vi "7. CoffeeMaker User Selection.vi"() -> ()   [LabVIEW 2018]
doc: "Coffee Machine Version 1.0: reacting correctly on user selections"
uses:
  Controls/States.ctl
  <vilib>/Utility/miscctls.llb/LVMinMaxIncTypeDef.ctl
  <vilib>/Utility/file.llb/Read Delimited Spreadsheet (string).vi
panel:
  out "s? t:f":enum16{"next state", "current state"}(ring)
  out "error out":errorcluster
  in  "error in (no error)":errorcluster
  in  "Power Switch":bool
  in  "Simulation":cluster{"Water":dbl, "Coffee":dbl, "Milk":dbl} caption="Wasser" {"Milk" scale=0.0..100.0; "Water" scale=0.0..100.0; "Coffee" scale=0.0..100.0}
  out "Display":T1 {"Coffee" scale=0.0..80.0; "Brewing Chamber" scale=0.0..80.0}
  in  "Coffee Selection":T2 {"Type" min=0 max=0 step=1 scale=0.0..2.0}
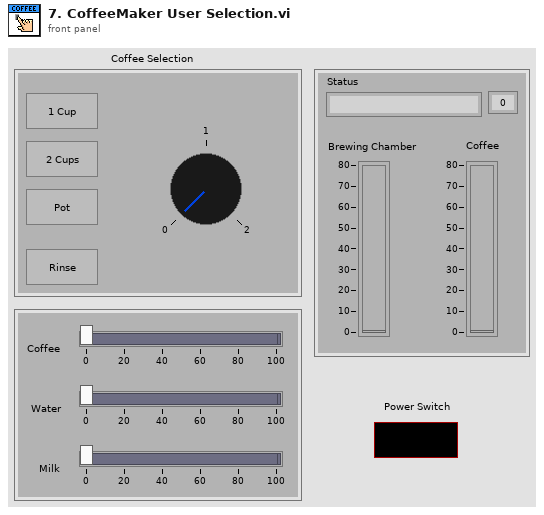
[diagram p1: front panel]
types:
  T1 = cluster{"Brewing Chamber":dbl, "Coffee":dbl, "Status":string, "Remaining Time:":i32}
  T2 = cluster{"1 Cup":bool, "2 Cups":bool, "Pot":bool, "Rinse":bool, "Type":i8}
  T3 = cluster{"Status":refnum<vi>, "Brewing Chamber":refnum<vi>, "Coffee":refnum<vi>, "Power Switch":refnum<vi>}
  T4 = enum8{"Enabled", "Disabled", "Disabled and Grayed Out"}
  T5 = typedef "LVMinMaxIncTypeDef.ctl" = cluster{"Minimum":dbl, "Maximum":dbl, "Increment":dbl}
  T6 = typedef "States.ctl" = enum16{"Initialize", "Set Language", "Wait for Power On", "Heat up", "Check and Wait for Water", "Rinsing", "Check Resources", "User Input", "Grinding", "Boiling", "Pouring", "Rinse before Stop", "Write Data", "Stop"}
  T7 = cluster{"Coffee":refnum<vi>, "Water":refnum<vi>, "Milk":refnum<vi>}
  T8 = cluster{"Coffee Selection":refnum<vi>, "1 Cup":refnum<vi>, "2 Cups":refnum<vi>, "Pot":refnum<vi>, "Rinse":refnum<vi>, "Type":refnum<vi>}
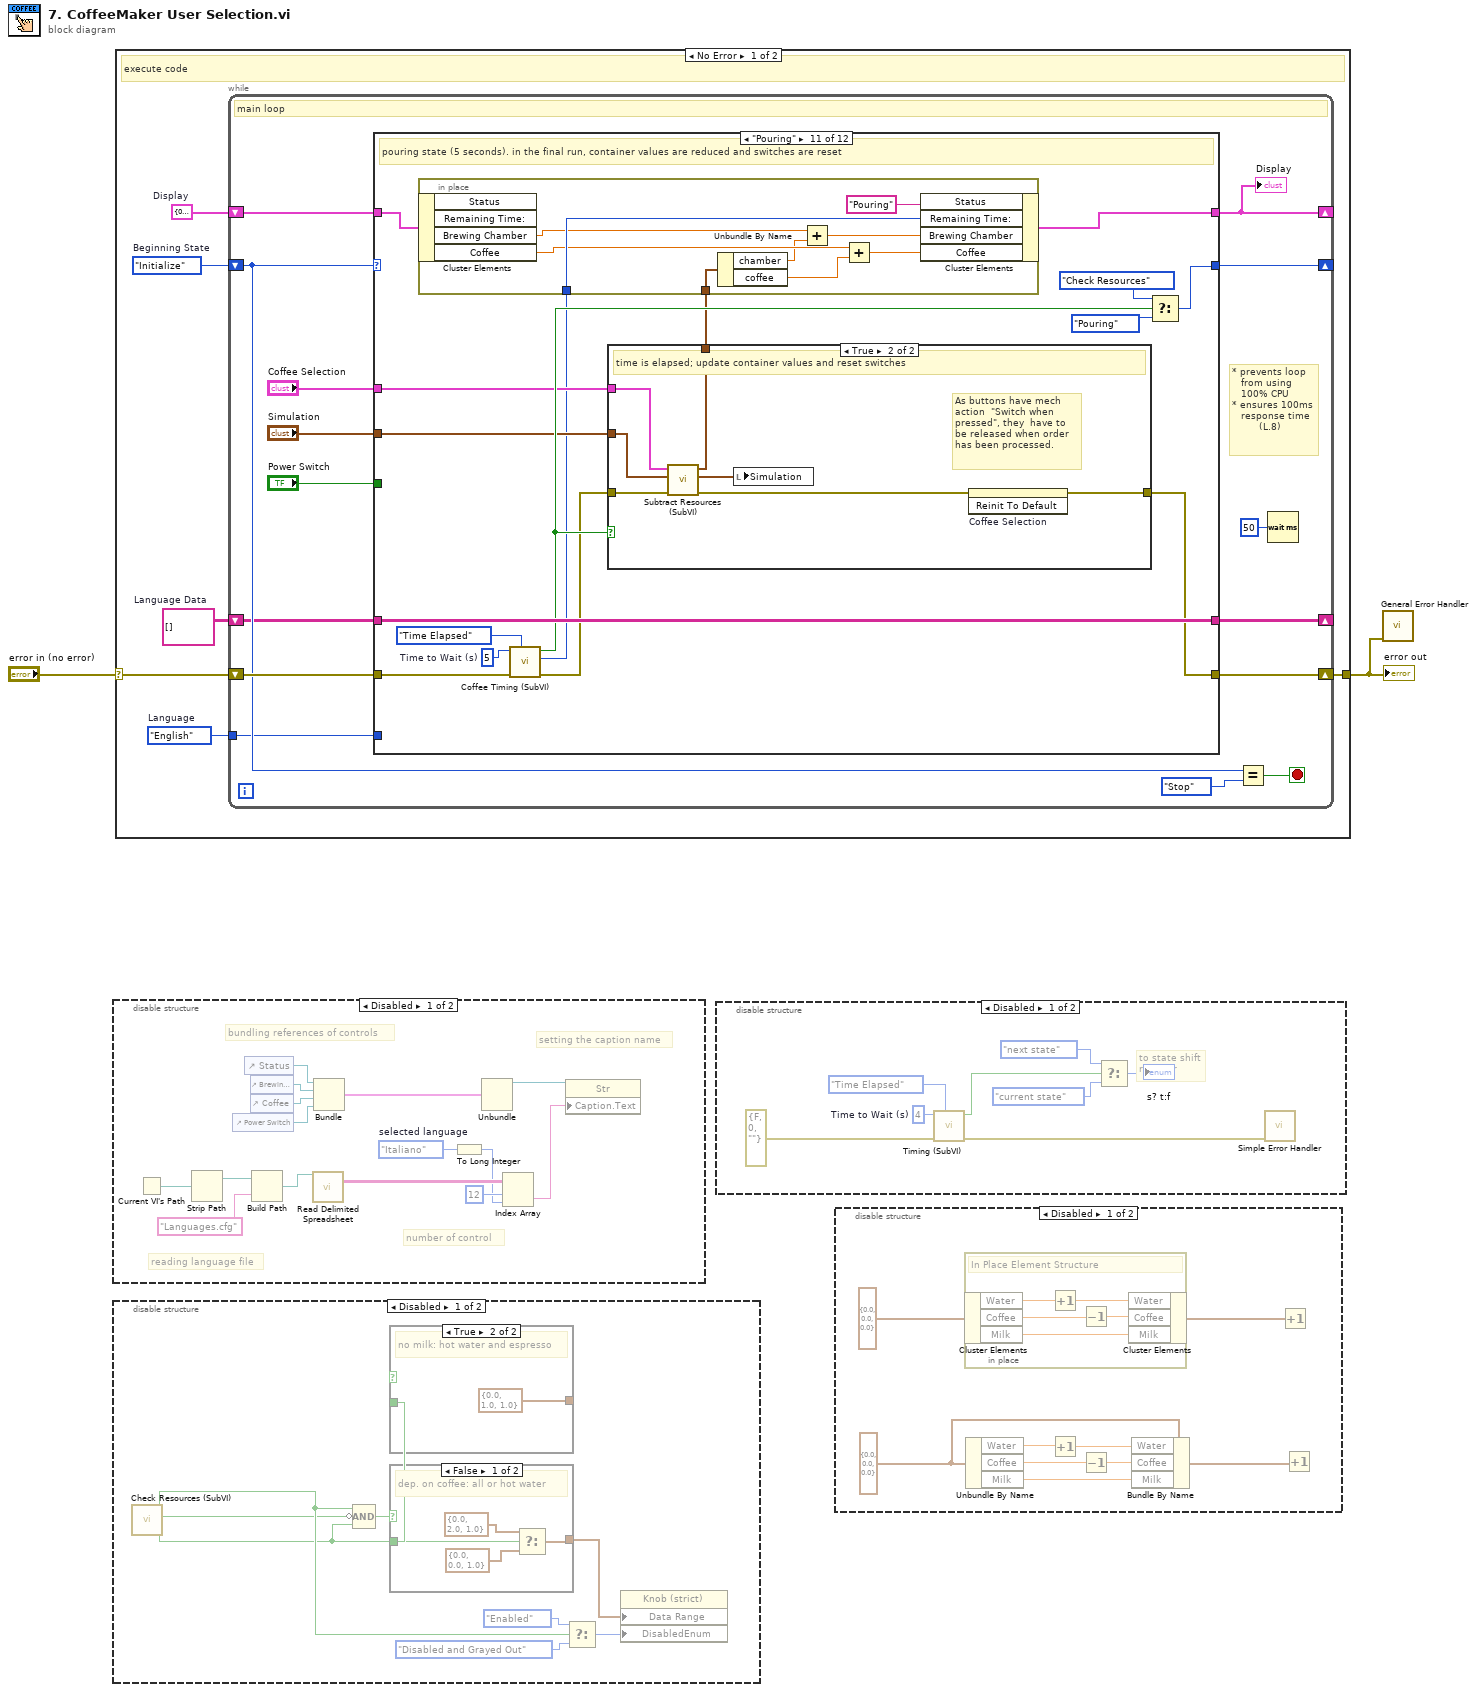
[diagram p0: block diagram]
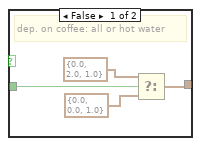
[diagram p3: hidden frame]
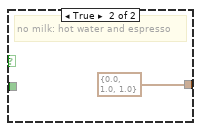
[diagram p4: hidden frame]
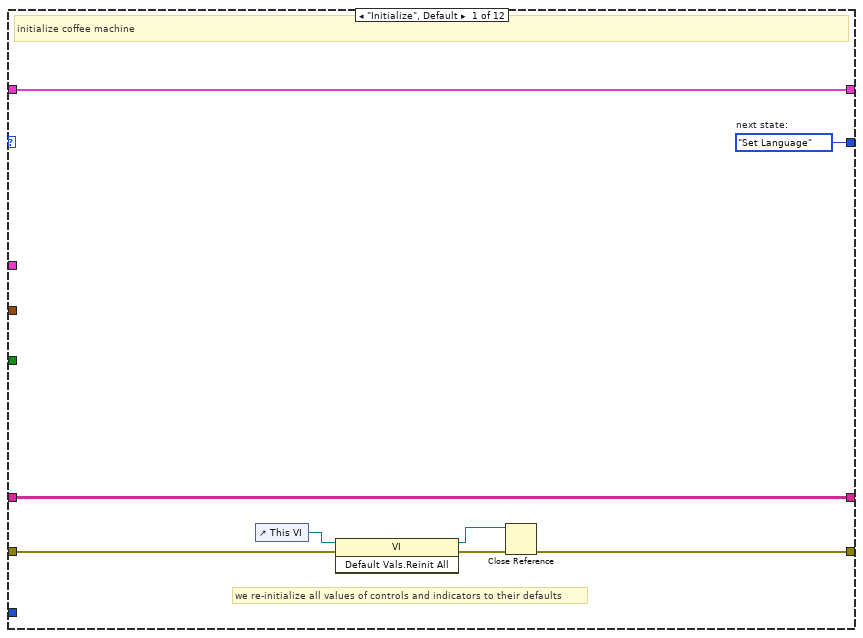
[diagram p8: hidden frame]
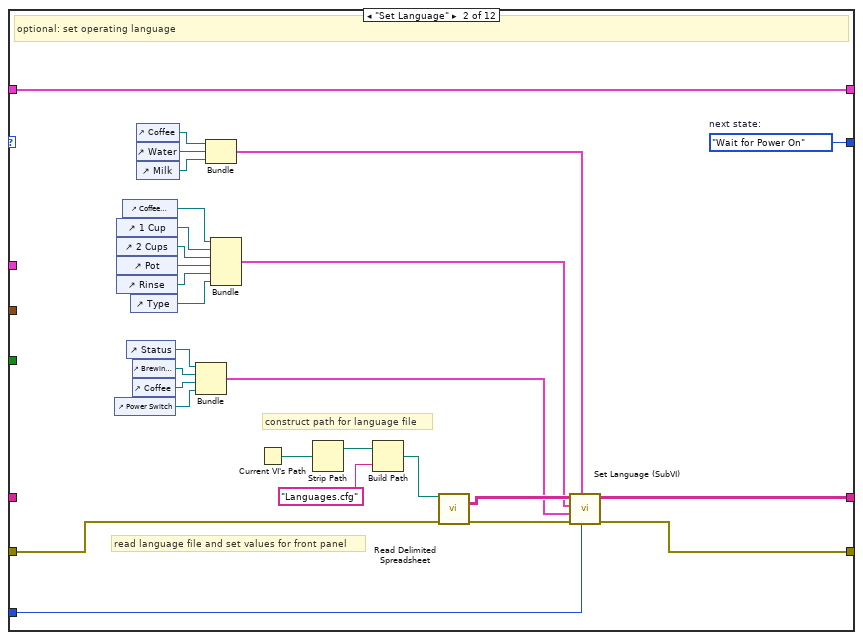
[diagram p9: hidden frame]
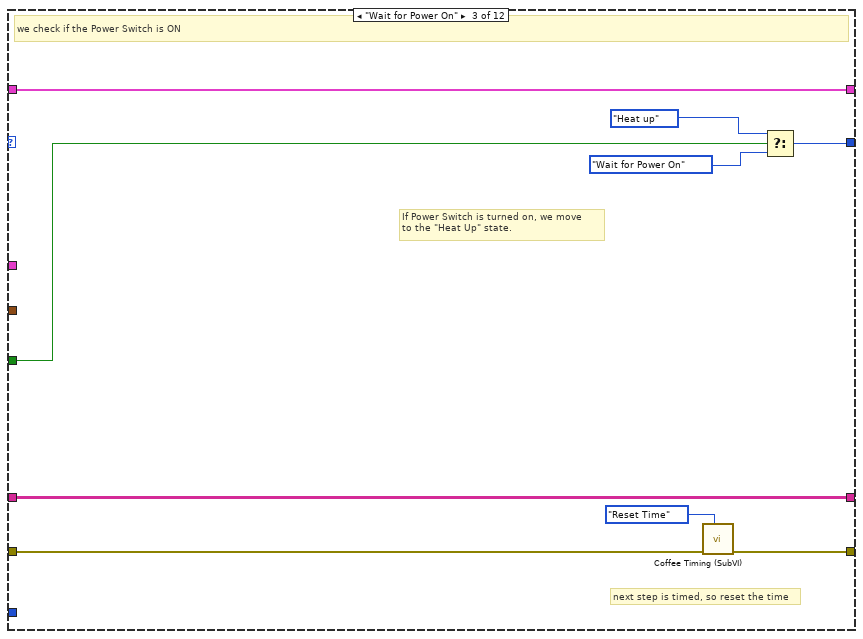
[diagram p10: hidden frame]
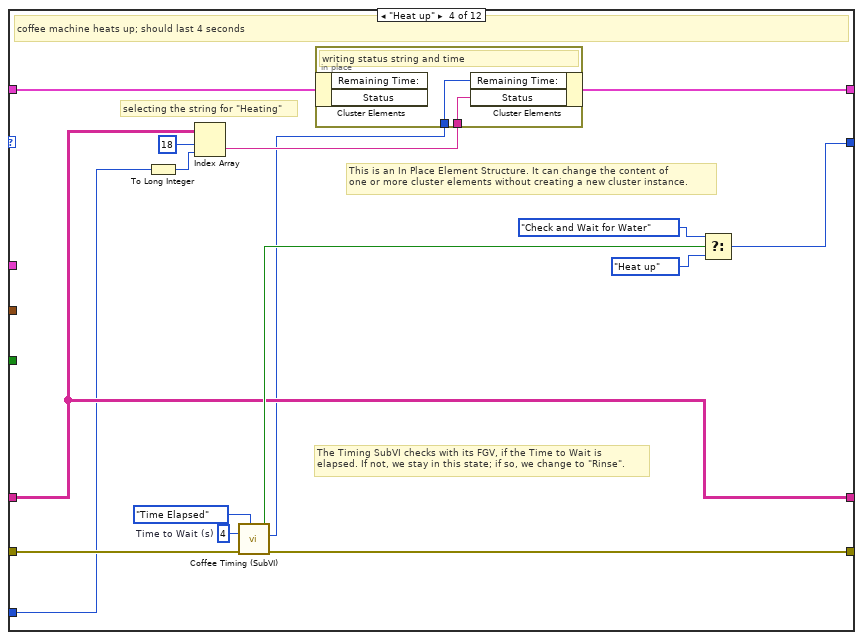
[diagram p11: hidden frame]
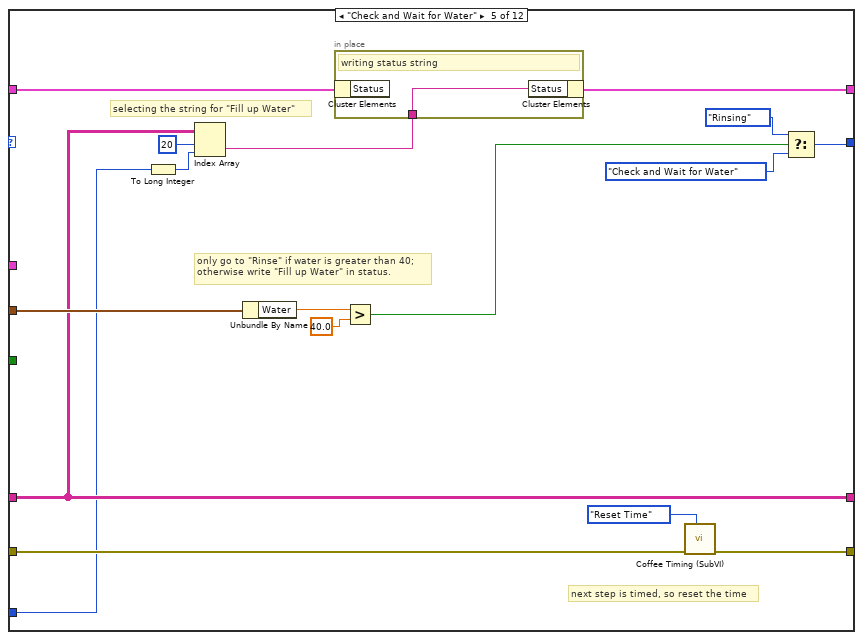
[diagram p12: hidden frame]
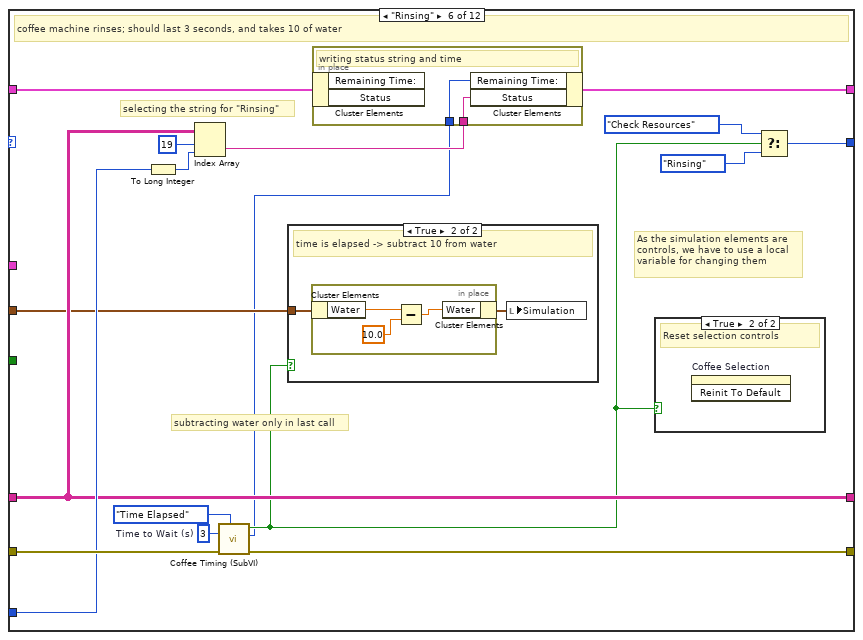
[diagram p13: hidden frame]
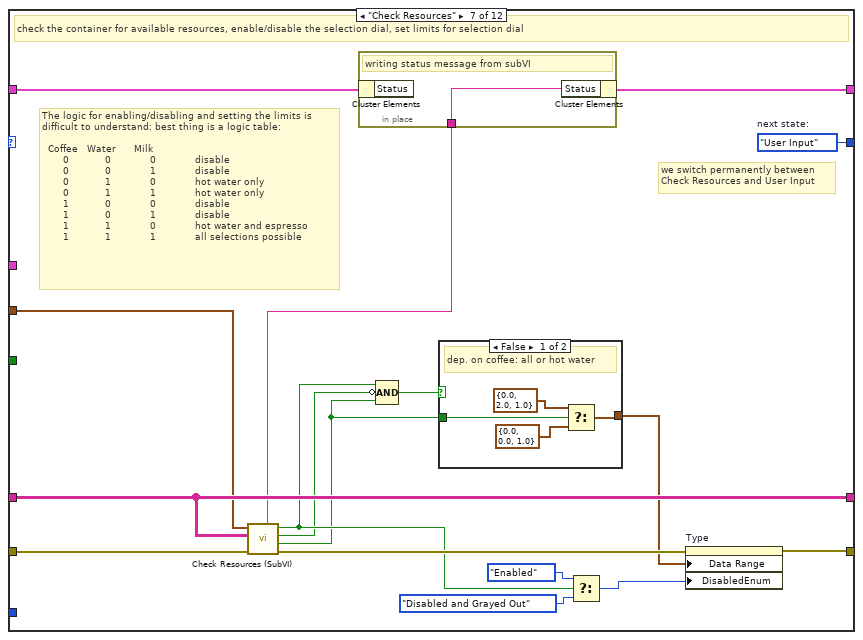
[diagram p16: hidden frame]
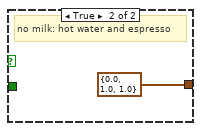
[diagram p17: hidden frame]
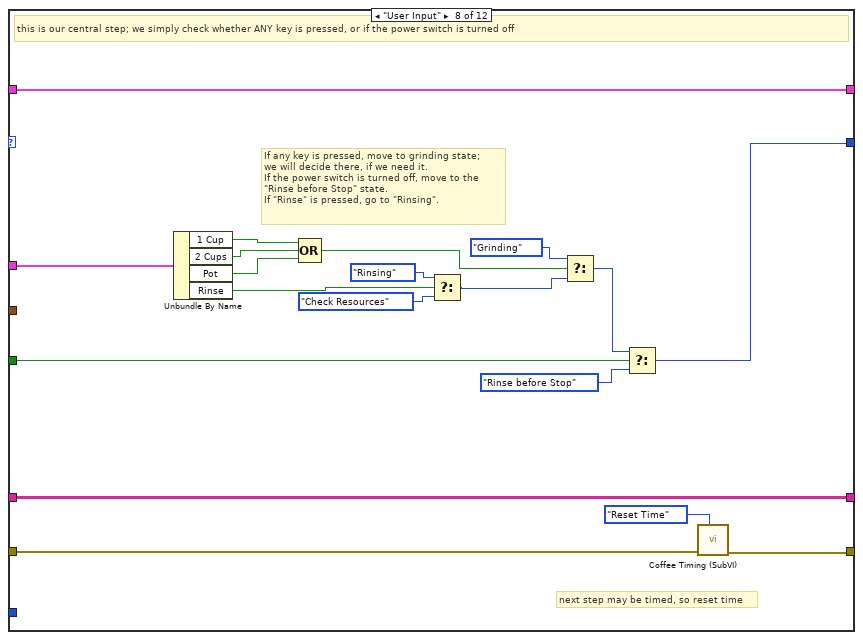
[diagram p18: hidden frame]
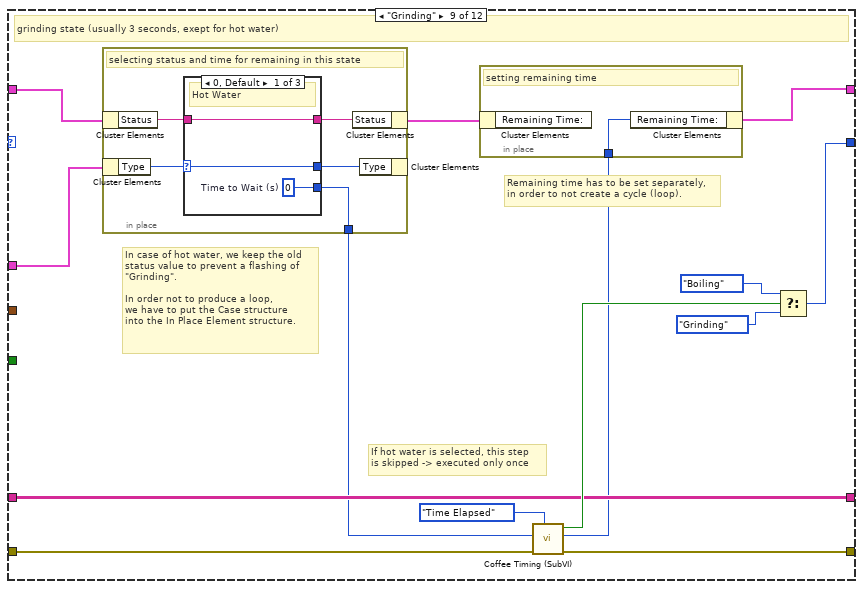
[diagram p19: hidden frame]
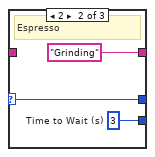
[diagram p20: hidden frame]
diagram:
  n1 = disable-structure shown="Disabled" {
    frame Disabled {
      w5 = enum16{"English", "Deutsch", "Italiano"}."Italiano"  # selected language
      # "setting the caption name"
      # "number of control"
      # "reading language file"
      # "bundling references of controls"
      n2 = Current VI's Path() -> (path=w11:path)
      n3 = Strip Path(path=w11) -> (stripped path=w10:path)  [unwired: 1 out]
      n4 = control-ref of="Power Switch"() -> (w17:refnum<vi>)
      n5 = control-ref of="Status"() -> (w14:refnum<vi>)
      n6 = control-ref of="Brewing Chamber"() -> (w15:refnum<vi>)
      n7 = control-ref of="Coffee"() -> (w16:refnum<vi>)
      n8 = Build Path(base path=w10, name or relative path="Languages.cfg") -> (appended path=w8:path)
      n9 = call-poly <vilib>:"Read Delimited Spreadsheet.vi"("file path (dialog if empty)"=w8) -> ("all rows"=w7:string[][])  [unwired: 9 in, 5 out]
      n10 = Bundle("Status"=w14, "Brewing Chamber"=w15, "Coffee"=w16, "Power Switch"=w17) -> (w13:T3)  [unwired: 1 in]
      n11 = To Long Integer(number=w5) -> (32bit integer=w4:i32)
      n12 = Unbundle(w13) -> ("Status"=w12:refnum<vi>)  [unwired: 3 out]
      n13 = Index Array(array=w7, index (row)=12, index (col)=w4) -> (element=w3:string)
      n14 = property class="Str"(reference=w12, "Caption.Text"=w3) -> ()  [unwired: 1 in, 2 out]
    }
    frame Enabled {
    }
  }
  n15 = disable-structure shown="Disabled" {
    frame Disabled {
      n16 = call "Check Resources (SubVI).vi"() -> ("Coffee ok?"=w18:bool, "Milk ok?"=w19:bool, "Water ok?"=w20:bool)  [unwired: 7 in, 2 out]
      n17 = Compound Arithmetic op=AND(w20, invert w19, w18) -> (w22:bool)
      n18 = case shown="True" {
        selector: _ -> [_ _]
        tunnel: w18 -> [w27 _]
        tunnel: [w26 T5 {"Minimum"=0.0, "Maximum"=1.0, "Increment"=1.0} ("Data Entry Limits")] -> _
        frame False {
          # "dep. on coffee: all or hot water"
          n19 = Select(t=T5 {"Minimum"=0.0, "Maximum"=2.0, "Increment"=1.0} ("Data Entry Limits"), s=w27, f=T5 {"Minimum"=0.0, "Maximum"=0.0, "Increment"=1.0} ("Data Entry Limits")) -> (s? t:f=w26:T5)
        }
        frame True {
          # "no milk: hot water and espresso"
        }
      }
      n20 = case shown="False" w22 {
        tunnel: w18 -> [w32 _]
        tunnel: [w31 T5 {"Minimum"=0.0, "Maximum"=1.0, "Increment"=1.0} ("Data Entry Limits")] -> w21
        frame False {
          # "dep. on coffee: all or hot water"
          n21 = Select(t=T5 {"Minimum"=0.0, "Maximum"=2.0, "Increment"=1.0} ("Data Entry Limits"), s=w32, f=T5 {"Minimum"=0.0, "Maximum"=0.0, "Increment"=1.0} ("Data Entry Limits")) -> (s? t:f=w31:T5)
        }
        frame True {
          # "no milk: hot water and espresso"
        }
      }
      n22 = Select(t=T4."Enabled" ("Disabled"), s=w20, f=T4."Disabled and Grayed Out" ("Disabled")) -> (s? t:f=w23:T4)
      n23 = property on="Property Node" class="Knob (strict)"("Data Range"=w21, "DisabledEnum"=w23) -> ()  [unwired: 2 in, 2 out]
    }
    frame Enabled {
    }
  }
  n24 = case shown="No Error" "error in (no error)" {
    selector: "error in (no error)" -> [w40 w308]
    tunnel: [w41 w308] -> w1
    frame No Error {
      w36 = T1 {"Brewing Chamber"=0.0, "Coffee"=0.0, "Status"="", "Remaining Time:"=0}  # Display
      w37 = enum16{"English", "Deutsch", "Italiano"}."English"  # Language
      w38 = string[][] []  # Language Data
      w39 = States."Initialize"  # Beginning State
      # "execute code"
      n25 = while {
        shift-right: [w53] -> _
        shift-left: w39 -> [w52]
        shift-right: [w46] -> _
        shift-left: w38 -> [w45]
        shift-right: [w42] -> _
        shift-left: w36 -> [w49]
        shift-right: [w56] -> w41
        shift-left: w40 -> [w55]
        tunnel: w37 -> [w43]
        stop <- w50 stop-if-true
        # "* prevents loop\n   from using\n   100% CPU\n* ensures 100ms\n   response time\n         (L.8)"
        # "main loop"
        n26 = case shown="\"Pouring\"" w52 {
          tunnel: [w58 w85 w96 w116 w127 w153 w168 w201 w215 w241 w249 w297] -> w56
          tunnel: w55 -> [w63 w86 w97 w117 w128 w154 w178 w202 w216 w242 w260 w298]
          tunnel: "Power Switch" -> [_ _ w101 _ _ _ _ w199 _ _ _ _]
          tunnel: [w60 w83 w100 w113 w134 w150 w172 w198 w212 w237 w257 w294] -> w53
          tunnel: [w59 w82 w94 w108 w120 w146 w173 w189 w204 w243 w261 w291] -> w42
          tunnel: w49 -> [w59 w82 w94 w109 w126 w147 w175 w189 w217 w244 w262 w292]
          tunnel: "Coffee Selection" -> [_ _ _ _ _ _ _ w197 w208 _ w251 _]
          tunnel: "Simulation" -> [_ _ _ _ w133 w140 w176 _ _ _ w252 w286]
          tunnel: [w57 w84 w93 w107 w123 w142 w177 w203 w209 w234 w254 w287] -> w46
          tunnel: w45 -> [w57 _ w93 w107 w123 w142 w177 w203 w209 w234 w254 w287]
          tunnel: w43 -> [_ w69 _ w104 w122 w143 _ _ _ _ _ w288]
          frame "Initialize", Default {
            w60 = States."Set Language"  # next state:
            # "we re-initialize all values of controls and indicators to their defaults"
            # "initialize coffee machine"
            n27 = control-ref of="This VI"() -> (w64:refnum<vi>)
            n28 = invoke class="VI" method="Default Vals.Reinit All"(reference=w64, error in=w63) -> (reference out=w62:refnum<vi>, error out=w61:errorcluster)  [unwired: 1 in, 1 out]
            n29 = Close Reference(reference=w62, error in (no error)=w61) -> (error out=w58:errorcluster)
          }
          frame "Set Language" {
            w83 = States."Wait for Power On"  # next state:
            # "construct path for language file"
            # "read language file and set values for front panel"
            # "optional: set operating language"
            n30 = control-ref of="Power Switch"() -> (w72:refnum<vi>)
            n31 = control-ref of="1 Cup"() -> (w80:refnum<vi>)
            n32 = control-ref of="2 Cups"() -> (w79:refnum<vi>)
            n33 = control-ref of="Pot"() -> (w78:refnum<vi>)
            n34 = control-ref of="Rinse"() -> (w77:refnum<vi>)
            n35 = control-ref of="Coffee Selection"() -> (w81:refnum<vi>)
            n36 = control-ref of="Status"() -> (w75:refnum<vi>)
            n37 = control-ref of="Type"() -> (w76:refnum<vi>)
            n38 = control-ref of="Brewing Chamber"() -> (w74:refnum<vi>)
            n39 = control-ref of="Coffee"() -> (w73:refnum<vi>)
            n40 = control-ref of="Coffee"() -> (w68:refnum<vi>)
            n41 = control-ref of="Water"() -> (w67:refnum<vi>)
            n42 = control-ref of="Milk"() -> (w66:refnum<vi>)
            n43 = Bundle("Status"=w75, "Brewing Chamber"=w74, "Coffee"=w73, "Power Switch"=w72) -> (w70:T3)  [unwired: 1 in]
            n44 = Bundle("Coffee"=w68, "Water"=w67, "Milk"=w66) -> (w65:T7)  [unwired: 1 in]
            n45 = Bundle("Coffee Selection"=w81, "1 Cup"=w80, "2 Cups"=w79, "Pot"=w78, "Rinse"=w77, "Type"=w76) -> (w71:T8)  [unwired: 1 in]
            n46 = Current VI's Path() -> (path=w87:path)
            n47 = Strip Path(path=w87) -> (stripped path=w88:path)  [unwired: 1 out]
            n48 = Build Path(base path=w88, name or relative path="Languages.cfg") -> (appended path=w90:path)
            n49 = call-poly <vilib>:"Read Delimited Spreadsheet.vi"("file path (dialog if empty)"=w90, "error in (no error)"=w86) -> ("all rows"=w92:string[][], "error out"=w91:errorcluster)  [unwired: 8 in, 4 out]
            n50 = call "Set Language (SubVI).vi"("Language (English)"=w69, "Simulation \nReferences"=w65, "error in (no error)"=w91, "Status\nReferences"=w70, "Selection \nReferences"=w71, "Language Data"=w92) -> ("error out"=w85:errorcluster, "Language Data Out"=w84:string[][])  [unwired: 4 in]
          }
          frame "Wait for Power On" {
            # "next step is timed, so reset the time"
            # "If Power Switch is turned on, we move\nto the \"Heat Up\" state."
            # "we check if the Power Switch is ON"
            n51 = call "Coffee Timing (SubVI).vi"("Function"=enum16{"Reset Time", "Time Elapsed"}."Reset Time", "error in (no error)"=w97) -> ("error out"=w96:errorcluster)  [unwired: 7 in, 2 out]
            n52 = Select(t=States."Heat up" ("Beginning State"), s=w101, f=States."Wait for Power On") -> (s? t:f=w100:T6)
          }
          frame "Heat up" {
            w114 = 4  # Time to Wait (s)
            # "selecting the string for \"Heating\""
            # "This is an In Place Element Structure. It can change the content of\none or more cluster elements without creating a new cluster instance."
            # "The Timing SubVI checks with its FGV, if the Time to Wait is\nelapsed. If not, we stay in this state; if so, we change to \"Rinse\"."
            # "coffee machine heats up; should last 4 seconds"
            n53 = To Long Integer(number=w104) -> (32bit integer=w105:i32)
            n54 = Index Array "Index Array"(array=w107, index (row)=18, index (col)=w105) -> (element=w103:string)
            n55 = call "Coffee Timing (SubVI).vi"("Function"=enum16{"Reset Time", "Time Elapsed"}."Time Elapsed", "error in (no error)"=w117, "Time to Wait (s)"=w114) -> ("error out"=w116:errorcluster, "Remaining Time"=w102:i32, "Time elapsed ?"=w110:bool)  [unwired: 6 in]
            n56 = in-place {
              in-place-border: w103 -> [w119]
              in-place-border: w102 -> [w118]
              # "writing status string and time"
              n57 = in-place-cluster #1(w109) -> ()  [unwired: 2 out]
              n58 = in-place-cluster #1("Remaining Time:"=w118, "Status"=w119) -> (w108:T1)
            }
            n59 = Select(t=States."Check and Wait for Water" ("Beginning State"), s=w110, f=States."Heat up" ("Beginning State")) -> (s? t:f=w113:T6)
          }
          frame "Check and Wait for Water" {
            # "next step is timed, so reset the time"
            # "only go to \"Rinse\" if water is greater than 40;\notherwise write \"Fill up Water\" in status."
            # "selecting the string for \"Fill up Water\""
            n60 = To Long Integer(number=w122) -> (32bit integer=w124:i32)
            n61 = Index Array "Index Array"(array=w123, index (row)=20, index (col)=w124) -> (element=w121:string)
            n62 = Unbundle By Name(w133) -> ("Water"=w132:dbl)
            n63 = in-place {
              in-place-border: w121 -> [w137]
              # "writing status string"
              n64 = in-place-cluster #2(w126) -> ()  [unwired: 1 out]
              n65 = in-place-cluster #2("Status"=w137) -> (w120:T1)
            }
            n66 = Greater?(x=w132, y=40.0) -> (0:w130:bool)
            n67 = call "Coffee Timing (SubVI).vi"("Function"=enum16{"Reset Time", "Time Elapsed"}."Reset Time", "error in (no error)"=w128) -> ("error out"=w127:errorcluster)  [unwired: 7 in, 2 out]
            n68 = Select(t=States."Rinsing" ("f"), s=w130, f=States."Check and Wait for Water") -> (s? t:f=w134:T6)
          }
          frame "Rinsing" {
            w151 = 3  # Time to Wait (s)
            # "subtracting water only in last call"
            # "As the simulation elements are\ncontrols, we have to use a local\nvariable for changing them"
            # "selecting the string for \"Rinsing\""
            # "coffee machine rinses; should last 3 seconds, and takes 10 of water"
            n69 = To Long Integer(number=w143) -> (32bit integer=w144:i32)
            n70 = Index Array "Index Array"(array=w142, index (row)=19, index (col)=w144) -> (element=w141:string)
            n71 = call "Coffee Timing (SubVI).vi"("Function"=enum16{"Reset Time", "Time Elapsed"}."Time Elapsed", "error in (no error)"=w154, "Time to Wait (s)"=w151) -> ("error out"=w153:errorcluster, "Remaining Time"=w138:i32, "Time elapsed ?"=w139:bool)  [unwired: 6 in]
            n72 = case shown="True" w139 {
              tunnel: w140 -> [_ w156]
              frame False {
                # "time is running ..."
              }
              frame True {
                # "time is elapsed -> subtract 10 from water"
                n73 = in-place {
                  n74 = in-place-cluster #3(w156) -> ("Water"=w159:dbl)
                  n75 = Subtract(x=w159, y=10.0) -> (x-y=w157:dbl)
                  n76 = in-place-cluster #3("Water"=w157) -> (w155:cluster{"Water":dbl, "Coffee":dbl, "Milk":dbl})
                }
                n77 = local write "Simulation"(w155) -> ()
              }
            }
            n78 = in-place {
              in-place-border: w141 -> [w161]
              in-place-border: w138 -> [w160]
              # "writing status string and time"
              n79 = in-place-cluster #4(w147) -> ()  [unwired: 2 out]
              n80 = in-place-cluster #4("Remaining Time:"=w160, "Status"=w161) -> (w146:T1)
            }
            n81 = case shown="True" w139 {
              frame False {
              }
              frame True {
                # "Reset selection controls"
                n82 = invoke on="Coffee Selection" class="Clust (strict)" method="Reinit To Default"() -> ()  [unwired: 3 in, 3 out]
              }
            }
            n83 = Select(t=States."Check Resources" ("Beginning State"), s=w139, f=States."Rinsing" ("Beginning State")) -> (s? t:f=w150:T6)
          }
          frame "Check Resources" {
            w172 = States."User Input"  # next state:
            # "The logic for enabling/disabling and setting the limits is \ndifficult to understand: best thing is a logic table:\n\n  Coffee   Water      Milk\n       0            0             0             disable\n       0            0             1             disable\n       0            1             0             hot water only\n       0            1             1             hot water only\n       1            0             0             disable\n       1            0             1             disable\n       1            1             0             hot water and espresso\n       1            1             1             all selections possible"
            # "we switch permanently between \nCheck Resources and User Input"
            # "check the container for available resources, enable/disable the selection dial, set limits for selection dial"
            n84 = call "Check Resources (SubVI).vi"("error in (no error)"=w178, "Language Data"=w177, "Simulation"=w176) -> ("error out"=w169:errorcluster, "Coffee ok?"=w163:bool, "Milk ok?"=w165:bool, "Water ok?"=w166:bool, "Status Message"=w174:string)  [unwired: 4 in]
            n85 = in-place {
              in-place-border: w174 -> [w184]
              # "writing status message from subVI"
              n86 = in-place-cluster #5(w175) -> ()  [unwired: 1 out]
              n87 = in-place-cluster #5("Status"=w184) -> (w173:T1)
            }
            n88 = Compound Arithmetic op=AND(w166, invert w165, w163) -> (w164:bool)
            n89 = case shown="False" w164 {
              tunnel: w163 -> [w180 _]
              tunnel: [w179 T5 {"Minimum"=0.0, "Maximum"=1.0, "Increment"=1.0} ("Data Entry Limits")] -> w162
              frame False {
                # "dep. on coffee: all or hot water"
                n90 = Select(t=T5 {"Minimum"=0.0, "Maximum"=2.0, "Increment"=1.0} ("Data Entry Limits"), s=w180, f=T5 {"Minimum"=0.0, "Maximum"=0.0, "Increment"=1.0} ("Data Entry Limits")) -> (s? t:f=w179:T5)
              }
              frame True {
                # "no milk: hot water and espresso"
              }
            }
            n91 = Select(t=T4."Enabled" ("Disabled"), s=w166, f=T4."Disabled and Grayed Out" ("Disabled")) -> (s? t:f=w167:T4)
            n92 = property on="Type" class="Knob (strict)"(error in=w169, "Data Range"=w162, "DisabledEnum"=w167) -> (error out=w168:errorcluster)  [unwired: 1 in, 1 out]
          }
          frame "User Input" {
            # "If any key is pressed, move to grinding state; \nwe will decide there, if we need it.\nIf the power switch is turned off, move to the \n\"Rinse before Stop\" state.\nIf \"Rinse\" is pressed, go to \"Rinsing\"."
            # "next step may be timed, so reset time"
            # "this is our central step; we simply check whether ANY key is pressed, or if the power switch is turned off"
            n93 = Unbundle By Name(w197) -> ("1 Cup"=w196:bool, "2 Cups"=w195:bool, "Pot"=w194:bool, "Rinse"=w188:bool)
            n94 = Compound Arithmetic op=OR(w196, w195, w194) -> (w191:bool)
            n95 = Select(t=States."Rinsing", s=w188, f=States."Check Resources" ("t")) -> (s? t:f=w185:T6)
            n96 = Select(t=States."Grinding", s=w191, f=w185) -> (s? t:f=w192:T6)
            n97 = Select(t=w192, s=w199, f=States."Rinse before Stop") -> (s? t:f=w198:T6)
            n98 = call "Coffee Timing (SubVI).vi"("Function"=enum16{"Reset Time", "Time Elapsed"}."Reset Time", "error in (no error)"=w202) -> ("error out"=w201:errorcluster)  [unwired: 7 in, 2 out]
          }
          frame "Grinding" {
            # "Remaining time has to be set separately,\nin order to not create a cycle (loop)."
            # "In case of hot water, we keep the old\nstatus value to prevent a flashing of\n\"Grinding\".\n\nIn order not to produce a loop,\nwe have to put the Case structure\ninto the In Place Element structure."
            # "If hot water is selected, this step\nis skipped -> executed only once"
            # "grinding state (usually 3 seconds, exept for hot water)"
            n99 = in-place {
              in-place-border: [w220] -> w207
              # "selecting status and time for remaining in this state"
              n100 = in-place-cluster #6(w217) -> ("Status"=w222:string)
              n101 = in-place-cluster #7(w208) -> ("Type"=w223:i8)
              n102 = case shown="0, Default" w223 {
                selector: w223 -> [w224 w227 w230]
                tunnel: [w226 w229 w232] -> w220
                tunnel: [w225 "Grinding" ("Status") "Grinding" ("Status")] -> w221
                tunnel: w222 -> [w225 _ _]
                tunnel: [w224 w227 w230] -> w219
                frame 0, Default {
                  w226 = 0  # Time to Wait (s)
                  # "Hot Water"
                }
                frame 2 {
                  w229 = 3  # Time to Wait (s)
                  # "Espresso"
                }
                frame 1 {
                  w232 = 3  # Time to Wait (s)
                  # "Coffee"
                }
              }
              n103 = in-place-cluster #6("Status"=w221) -> (w206:T1)
              n104 = in-place-cluster #7("Type"=w219) -> ()  [unwired: 1 out]
            }
            n105 = call "Coffee Timing (SubVI).vi"("Function"=enum16{"Reset Time", "Time Elapsed"}."Time Elapsed", "error in (no error)"=w216, "Time to Wait (s)"=w207) -> ("error out"=w215:errorcluster, "Remaining Time"=w205:i32, "Time elapsed ?"=w213:bool)  [unwired: 6 in]
            n106 = in-place {
              in-place-border: w205 -> [w218]
              # "setting remaining time"
              n107 = in-place-cluster #8(w206) -> ()  [unwired: 1 out]
              n108 = in-place-cluster #8("Remaining Time:"=w218) -> (w204:T1)
            }
            n109 = Select(t=States."Boiling" ("Beginning State"), s=w213, f=States."Grinding") -> (s? t:f=w212:T6)
          }
          frame "Boiling" {
            w240 = 3  # Time to Wait (s)
            # "nothing special happens here"
            # "boiling state (3 seconds)"
            n110 = call "Coffee Timing (SubVI).vi"("Function"=enum16{"Reset Time", "Time Elapsed"}."Time Elapsed", "error in (no error)"=w242, "Time to Wait (s)"=w240) -> ("error out"=w241:errorcluster, "Remaining Time"=w233:i32, "Time elapsed ?"=w238:bool)  [unwired: 6 in]
            n111 = in-place {
              in-place-border: w233 -> [w245]
              n112 = in-place-cluster #9(w244) -> ()  [unwired: 2 out]
              n113 = in-place-cluster #9("Status"="Boiling", "Remaining Time:"=w245) -> (w243:T1)
            }
            n114 = Select(t=States."Pouring" ("Beginning State"), s=w238, f=States."Boiling") -> (s? t:f=w237:T6)
          }
          frame "Pouring" {
            w259 = 5  # Time to Wait (s)
            # "pouring state (5 seconds). in the final run, container values are reduced and switches are reset"
            n115 = call "Coffee Timing (SubVI).vi"("Function"=enum16{"Reset Time", "Time Elapsed"}."Time Elapsed", "error in (no error)"=w260, "Time to Wait (s)"=w259) -> ("error out"=w250:errorcluster, "Remaining Time"=w248:i32, "Time elapsed ?"=w253:bool)  [unwired: 6 in]
            n116 = case shown="True" w253 {
              tunnel: w252 -> [_ w270]
              tunnel: w251 -> [_ w271]
              tunnel: w250 -> [w264 w268]
              tunnel: [w264 w266] -> w249
              tunnel: [cluster{"coffee":dbl, "chamber":dbl} {"coffee"=0.0, "chamber"=0.0} ("Coffe and Chamber increase") w265] -> w247
              frame False {
                # "... time is still running ..."
              }
              frame True {
                # "As buttons have mech \naction  \"Switch when \npressed\", they  have to \nbe released when order \nhas been processed."
                # "time is elapsed; update container values and reset switches"
                n117 = call "Subtract Resources (SubVI).vi"("error in (no error)"=w268, "Simulation in"=w270, "Coffee Selection"=w271) -> ("error out"=w267:errorcluster, "Simulation out"=w269:cluster{"Water":dbl, "Coffee":dbl, "Milk":dbl}, "Coffe and Chamber increase"=w265:cluster{"coffee":i8, "chamber":i8})  [unwired: 6 in]
                n118 = local write "Simulation"(w269) -> ()
                n119 = invoke on="Coffee Selection" class="Clust (strict)" method="Reinit To Default"(error in=w267) -> (error out=w266:errorcluster)  [unwired: 2 in, 2 out]
              }
            }
            n120 = in-place {
              in-place-border: w248 -> [w279]
              in-place-border: w247 -> [w278]
              n121 = in-place-cluster #10(w262) -> ("Brewing Chamber"=w277:dbl, "Coffee"=w275:dbl)  [unwired: 2 out]
              n122 = Unbundle By Name(w278) -> ("chamber"=w272:dbl, "coffee"=w273:dbl)
              n123 = Add(x=w277, y=w272) -> (x+y=w276:dbl)
              n124 = Add(x=w275, y=w273) -> (x+y=w274:dbl)
              n125 = in-place-cluster #10("Status"="Pouring", "Remaining Time:"=w279, "Brewing Chamber"=w276, "Coffee"=w274) -> (w261:T1)
            }
            n126 = Select(t=States."Check Resources" ("Beginning State"), s=w253, f=States."Pouring") -> (s? t:f=w257:T6)
          }
          frame "Rinse before Stop" {
            w295 = 3  # Time to Wait (s)
            # "subtracting water only in last call"
            # "selecting the string for \"Rinsing\""
            # "coffee machine rinses before stopping; should last 3 seconds, and takes 10 of water"
            n127 = To Long Integer(number=w288) -> (32bit integer=w289:i32)
            n128 = Index Array "Index Array"(array=w287, index (row)=19, index (col)=w289) -> (element=w282:string)
            n129 = call "Coffee Timing (SubVI).vi"("Function"=enum16{"Reset Time", "Time Elapsed"}."Time Elapsed", "error in (no error)"=w298, "Time to Wait (s)"=w295) -> ("error out"=w297:errorcluster, "Remaining Time"=w281:i32, "Time elapsed ?"=w284:bool)  [unwired: 6 in]
            n130 = case shown="True" w284 {
              tunnel: [w299 ""] -> w283
              tunnel: w282 -> [w299 _]
              frame False {
                # "write status"
              }
              frame True {
                # "clear status"
              }
            }
            n131 = in-place {
              in-place-border: w283 -> [w307]
              in-place-border: w281 -> [w306]
              # "writing status string"
              n132 = in-place-cluster #11(w292) -> ()  [unwired: 2 out]
              n133 = in-place-cluster #11("Status"=w307, "Remaining Time:"=w306) -> (w291:T1)
            }
            n134 = case shown="True" w284 {
              tunnel: w286 -> [_ w302]
              frame False {
                # "time is running ..."
              }
              frame True {
                # "time is elapsed -> subtract 10 from water"
                n135 = in-place {
                  n136 = in-place-cluster #12(w302) -> ("Water"=w305:dbl)
                  n137 = Subtract(x=w305, y=10.0) -> (x-y=w303:dbl)
                  n138 = in-place-cluster #12("Water"=w303) -> (w301:cluster{"Water":dbl, "Coffee":dbl, "Milk":dbl})
                }
                n139 = local write "Simulation"(w301) -> ()
              }
            }
            n140 = Select(t=States."Stop" ("Beginning State"), s=w284, f=States."Rinse before Stop") -> (s? t:f=w294:T6)
          }
        }
        "Display" <- w42
        n141 = Equal?(x=w52, y=States."Stop") -> (x = y?=w50:bool)
        n142 = Wait (ms)(milliseconds to wait=u32 50) -> ()  [unwired: 1 out]
      }
    }
    frame Error {
      # "do nothing"
    }
  }
  "error out" <- w1
  n143 = disable-structure shown="Disabled" {
    frame Disabled {
      w315 = 4  # Time to Wait (s)
      # "to state shift\nregister"
      n144 = call "Timing (SubVI).vi"("Function"=enum16{"Reset Time", "Time Elapsed"}."Time Elapsed", "error in (no error)"=errorcluster {"status"=FALSE, "code"=0, "source"=""}, "Time to Wait (s)"=w315) -> ("error out"=w313:errorcluster, "Time elapsed ?"=w312:bool)  [unwired: 6 in, 1 out]
      n145 = Select(t=enum16{"next state", "current state"}."next state", s=w312, f=enum16{"next state", "current state"}."current state") -> (s? t:f=→"s? t:f":enum16{"next state", "current state"})
      n146 = call <vilib>:"Simple Error Handler.vi"("error in (no error)"=w313) -> ()  [unwired: 4 in, 5 out]
    }
    frame Enabled {
    }
  }
  n147 = disable-structure shown="Disabled" {
    frame Disabled {
      w323 = cluster{"Water":dbl, "Coffee":dbl, "Milk":dbl} {"Water"=0.0, "Coffee"=0.0, "Milk"=0.0} ("Simulation")
      n148 = in-place {
        # "In Place Element Structure"
        n149 = in-place-cluster #13(cluster{"Water":dbl, "Coffee":dbl, "Milk":dbl} {"Water"=0.0, "Coffee"=0.0, "Milk"=0.0} ("Simulation")) -> ("Water"=w330:dbl, "Coffee"=w328:dbl, "Milk"=w326:dbl)
        n150 = Increment(x=w330) -> (x+1=w329:dbl)
        n151 = Decrement(x=w328) -> (x-1=w327:dbl)
        n152 = in-place-cluster #13("Water"=w329, "Coffee"=w327, "Milk"=w326) -> (w324:cluster{"Water":dbl, "Coffee":dbl, "Milk":dbl})
      }
      n153 = Unbundle By Name(w323) -> ("Water"=w322:dbl, "Coffee"=w319:dbl, "Milk"=w318:dbl)
      n154 = Increment(x=w322) -> (x+1=w321:dbl)
      n155 = Decrement(x=w319) -> (x-1=w320:dbl)
      n156 = Bundle By Name(cluster=w323, "Water"=w321, "Coffee"=w320, "Milk"=w318) -> (w317:cluster{"Water":dbl, "Coffee":dbl, "Milk":dbl})
      n157 = Increment(x=w324) -> ()  [unwired: 1 out]
      n158 = Increment(x=w317) -> ()  [unwired: 1 out]
    }
    frame Enabled {
    }
  }
  n159 = call <vilib>:"General Error Handler.vi"("error in (no error)"=w1) -> ()  [unwired: 10 in, 5 out]
